vi "Process Return Value.vi"(10 "Method VI":refnum<vi>, 11 "QObject Writer in":refnum<class "QObject Writer.lvclass">) -> (2 "Modified Proto Method  VI":refnum<vi>, 3 "QObject Writer out":refnum<class "QObject Writer.lvclass">)   [LabVIEW 2013, in "QObject Writer.lvclass"]
uses:
  QObject Writer.lvclass
  Abstract Param Writer/Abstract Param Writer.lvclass
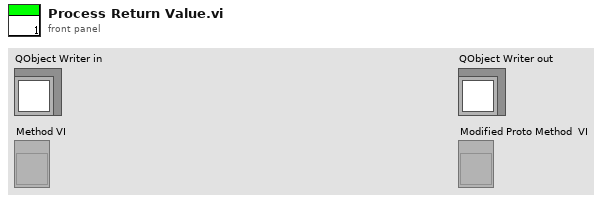
[diagram p1: front panel]
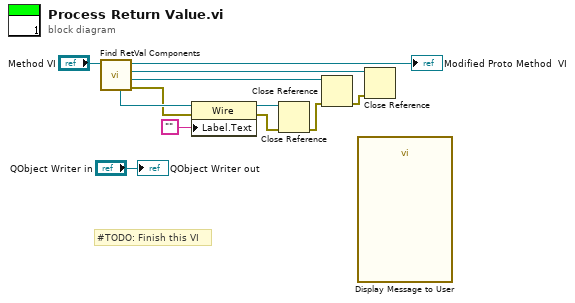
[diagram p0: block diagram]
diagram:
  # "#TODO: Finish this VI"
  n1 = call "Find RetVal Components.vi"("Proto Method VI"="Method VI") -> ("Error Out"=w10:errorcluster, "Indicator"=w6:refnum<vi>, "Data Buffer"=w4:refnum<vi>, "Proto Method VI Dup"=→"Modified Proto Method  VI":refnum<vi>, "Wire"=w12:refnum<vi>)  [unwired: 6 in]
  n2 = property class="Wire"(reference=w12, error in=w10, "Label.Text"="") -> (reference out=w8:refnum<vi>, error out=w9:errorcluster)
  n3 = Close Reference(reference=w8, error in (no error)=w9) -> (error out=w7:errorcluster)
  n4 = Close Reference(reference=w6, error in (no error)=w7) -> (error out=w5:errorcluster)
  n5 = call "Display Message to User"() -> ()  [unwired: 10 in, 2 out]
  n6 = Close Reference(reference=w4, error in (no error)=w5) -> ()  [unwired: 1 out]
  "QObject Writer out" <- "QObject Writer in"
